vi "S2DS_Change directionWCFromFile.vi"(7 "WC info list in":T1, 8 "Scan parameters  in":T3 {"Y data taking" items=["in both direction", "in up direction only", "in down direction only"]; "X data taking" items=["in both direction", "in up direction only", "in down direction only"]}, 9 "Y sweep direction":refnum<vi>, 10 "X sweep direction":refnum<vi>) -> (1 "Scan parameters out":T3 {"Y data taking" items=["in both direction", "in up direction only", "in down direction only"]; "X data taking" items=["in both direction", "in up direction only", "in down direction only"]}, 2 "Change color":bool)   [LabVIEW 2025]
uses:
  TYPE DEFS/S2DS_Sweep Info.ctl
  TYPE DEFS/S2DS_WC info.ctl
  TYPE DEFS/S2DS_Single WC info.ctl
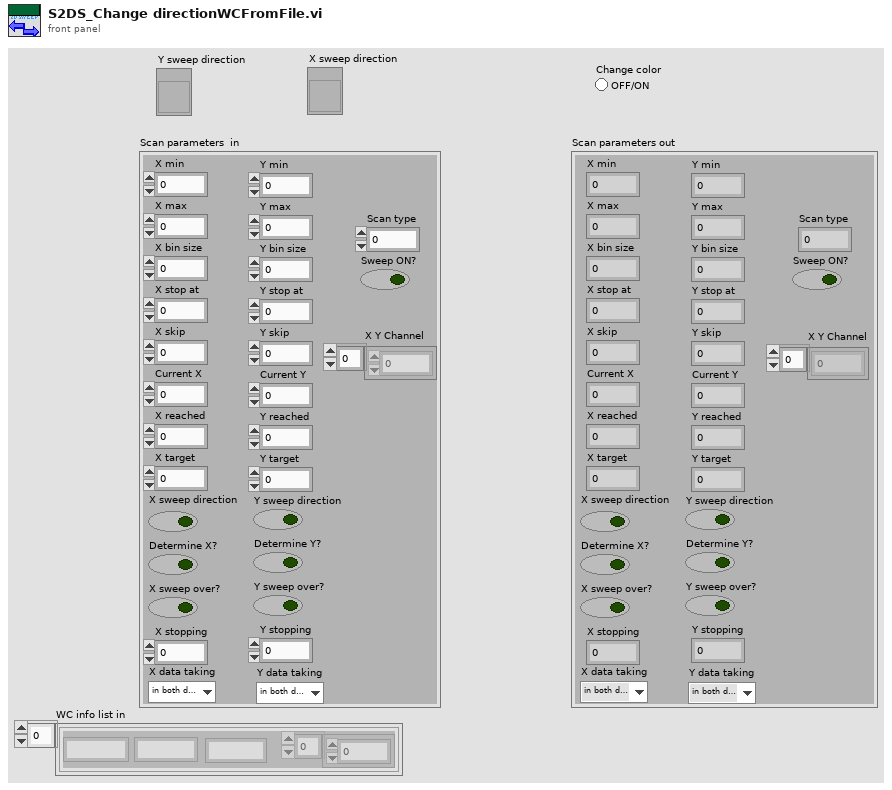
[diagram p1: front panel]
types:
  T1 = typedef "S2DS_WC info.ctl" = T2[]
  T2 = typedef "S2DS_Single WC info.ctl" = cluster{"Instrument identifier":string, "Write channel parameters":dbl[], "Name":string, "Unit":string}
  T3 = typedef "S2DS_Sweep Info.ctl" = cluster{"X min":ext, "X max":dbl, "Y min":dbl, "Y max":dbl, "X bin size":dbl, "Y bin size":dbl, "X stop at":dbl, "Y stop at":dbl, "X skip":u64, "Y skip":u64, "Current X":dbl, "Current Y":dbl, "X reached":i32, "Y reached":i32, "X target":dbl, "Y target":dbl, "Sweep ON?":bool, "X sweep direction":bool, "Y sweep direction":bool, "Determine X?":bool, "Determine Y?":bool, "X sweep over?":bool, "Y sweep over?":bool, "Scan type":i32, "X stopping":i32, "Y stopping":i32, "X Y Channel":u16[], "X data taking":u16, "Y data taking":u16}
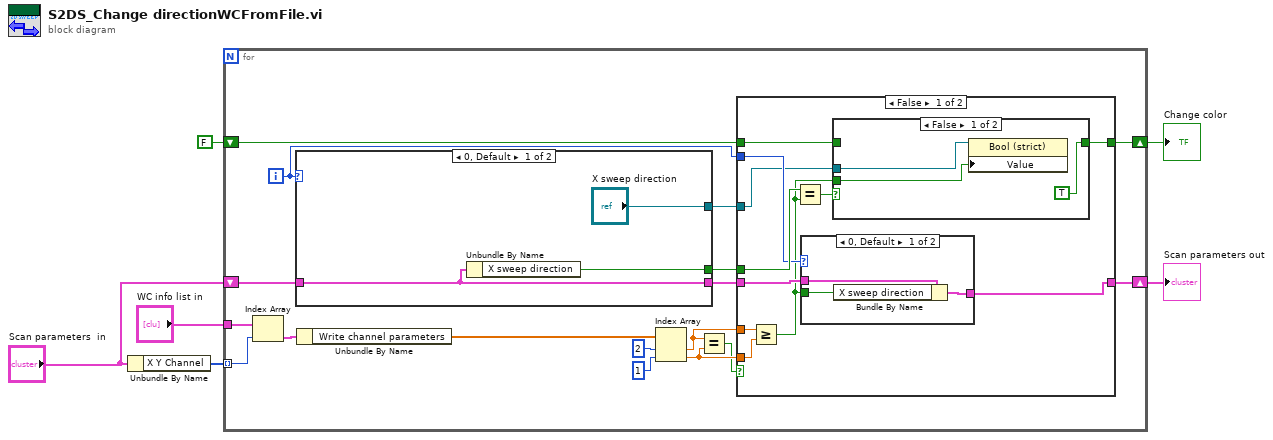
[diagram p0: block diagram]
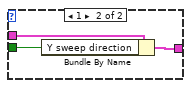
[diagram p3: hidden frame]
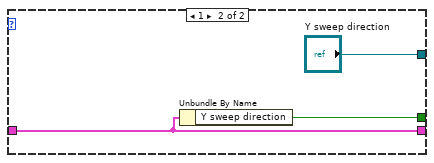
[diagram p5: hidden frame]
diagram:
  n1 = Unbundle By Name("Scan parameters  in") -> ("X Y Channel"=w6:u16[])
  n2 = for {
    tunnel: w6 -> [w22] mode=indexing
    tunnel: "WC info list in" -> [w23]
    shift-right: [w13] -> w3
    shift-left: "Scan parameters  in" -> [w17]
    shift-right: [w12] -> w1
    shift-left: FALSE -> [w11]
    i -> [w15]
    n3 = Index Array(array=w23, index=w22) -> (element=w21:T2)
    n4 = case shown="0, Default" w15 {
      tunnel: ["X sweep direction" "Y sweep direction"] -> w10
      tunnel: w17 -> [w47 w50]
      tunnel: [w48 w51] -> w16
      tunnel: [w47 w50] -> w14
      frame 0, Default {
        n5 = Unbundle By Name(w47) -> ("X sweep direction"=w48:bool)
      }
      frame 1 {
        n6 = Unbundle By Name(w50) -> ("Y sweep direction"=w51:bool)
      }
    }
    n7 = Unbundle By Name(w21) -> ("Write channel parameters"=w20:dbl[])
    n8 = Index Array(array=w20, index #1=2 ("index"), index #2=1 ("index")) -> (element #1=w8:dbl, element #2=w9:dbl)
    n9 = Equal?(x=w8, y=w9) -> (x = y?=w7:bool)
    n10 = case shown="False" w7 {
      tunnel: w8 -> [w34 _]
      tunnel: w9 -> [w33 _]
      tunnel: w16 -> [w32 _]
      tunnel: w15 -> [w31 _]
      tunnel: w14 -> [w30 w46]
      tunnel: [w29 w46] -> w13
      tunnel: [w27 w45] -> w12
      tunnel: w11 -> [w26 w45]
      tunnel: w10 -> [w24 _]
      frame False {
        n11 = Greater Or Equal?(x=w34, y=w33) -> (x >= y?=w25:bool)
        n12 = Equal?(x=w32, y=w25) -> (x = y?=w28:bool)
        n13 = case shown="0, Default" w31 {
          tunnel: w30 -> [w40 w44]
          tunnel: [w41 w43] -> w29
          tunnel: w25 -> [w39 w42]
          frame 0, Default {
            n14 = Bundle By Name(cluster=w40, "X sweep direction"=w39) -> (w41:T3)
          }
          frame 1 {
            n15 = Bundle By Name(cluster=w44, "Y sweep direction"=w42) -> (w43:T3)
          }
        }
        n16 = case shown="False" w28 {
          tunnel: [TRUE w38] -> w27
          tunnel: w26 -> [_ w38]
          tunnel: w25 -> [w36 _]
          tunnel: w24 -> [w35 _]
          frame False {
            n17 = property on="Property Node" class="Bool (strict)"(reference=w35, "Value"=w36) -> ()  [unwired: 1 in, 2 out]
          }
          frame True {
          }
        }
      }
      frame True {
      }
    }
  }
  "Scan parameters out" <- w3
  "Change color" <- w1
